vi "Write Description map.vi"(8 "error in (no error)":errorcluster, 10 "Description map":map{string, string}(c390), 11 "Test Tree in":refnum<class "Test Tree.lvclass">) -> (0 "error out":errorcluster, 3 "Test Tree out":refnum<class "Test Tree.lvclass">)   [LabVIEW 2020, in "Test Tree.lvclass"]
uses:
  Test Tree.lvclass
  Test Tree.lvclass/Test Tree.ctl
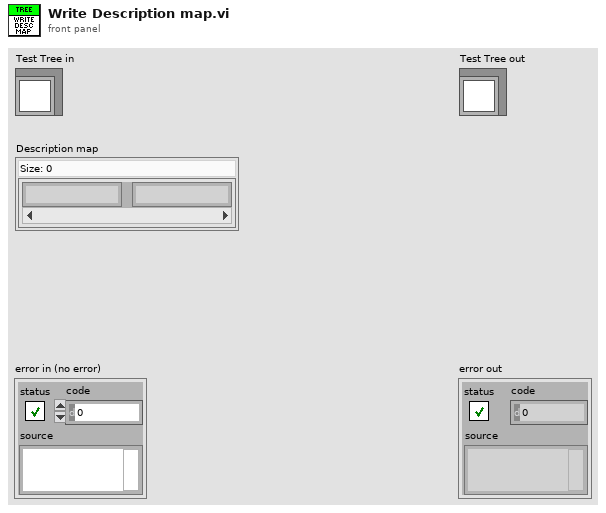
[diagram p1: front panel]
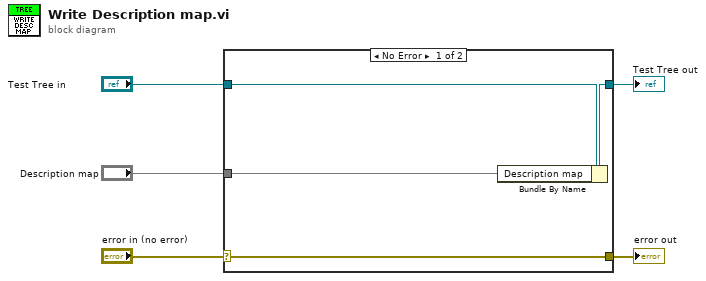
[diagram p0: block diagram]
diagram:
  n1 = case shown="No Error" "error in (no error)" {
    selector: "error in (no error)" -> [w9 w10]
    tunnel: [w9 w10] -> w4
    tunnel: [w7 w11] -> w2
    tunnel: "Test Tree in" -> [w8 w11]
    tunnel: "Description map" -> [w6 _]
    frame No Error {
      n2 = Bundle By Name(cluster=w8, "Description map"=w6) -> (w7:refnum<class "Test Tree.lvclass">)
    }
    frame Error {
    }
  }
  "error out" <- w4
  "Test Tree out" <- w2
